vi "save_spectroscopy_hdf.vi"(8 "Spectroscopy cluster in":T1, 11 "file path":path) -> ()   [LabVIEW 2019]
uses:
  <vilib>/UPVI/lvhdf5/file.llb/LVH5F Operation.ctl
  <vilib>/Utility/miscctls.llb/LVRectTypeDef.ctl
  <vilib>/UPVI/lvhdf5/group.llb/H5G_obj_t.ctl
  <vilib>/UPVI/lvhdf5/dataset.llb/LVH5D Operation.ctl
  <vilib>/UPVI/lvhdf5/attribute.llb/LVH5A Operation.ctl
  <vilib>/UPVI/lvhdf5/identifier.llb/Not an HDF5 Refnum Constant.vi
  <vilib>/UPVI/lvhdf5/common.llb/To HDF5 Ref.vi
  global_variables.vi
  <vilib>/UPVI/lvhdf5/attribute.llb/Write Multiple Attributes.vi
  <vilib>/UPVI/lvhdf5/utility.llb/Select HDF5 Dialog.vi
  <vilib>/UPVI/lvhdf5/utility.llb/Select HDF5 Dialog (Object Only).vi
  <vilib>/UPVI/lvhdf5/dataset.llb/Simple H5Dwrite (Variant).vi
  <vilib>/UPVI/lvhdf5/dataset.llb/H5Dclose.vi
  <vilib>/UPVI/lvhdf5/attribute.llb/Simple H5Awrite (Variant).vi
  <vilib>/UPVI/lvhdf5/attribute.llb/LVH5 Write Attributes.xnode
  <vilib>/UPVI/lvhdf5/library.llb/HDF5 Ref.ctl
  <vilib>/UPVI/lvhdf5/dataset.llb/Simple H5Dwrite.xnode
  <vilib>/UPVI/lvhdf5/dataset.llb/Write Dataset with Attributes.xnode
  <vilib>/UPVI/lvhdf5/attribute.llb/Simple H5Awrite.xnode
  <vilib>/Utility/VariantDataType/GetClusterInfo.vi
  <vilib>/Utility/VariantDataType/VariantType.lvlib
  <vilib>/Utility/VariantDataType/GetTypeInfo.vi
  <vilib>/UPVI/lvhdf5/attribute.llb/Cluster to Attribute Array.xnode
  <vilib>/Utility/error.llb/Error Cluster From Error Code.vi
  <vilib>/UPVI/lvhdf5/dataset.llb/OpenCreateReplace Dataset by Element Type.vi
  <vilib>/UPVI/lvhdf5/dataspace.llb/H5Sselect_hyperslab.vi
  <vilib>/UPVI/lvhdf5/dataset.llb/H5Dwrite (Variant).vi
  <vilib>/UPVI/lvhdf5/dataset.llb/H5Dget_space.vi
  <vilib>/UPVI/lvhdf5/attribute.llb/private/LVH5AwriteWDTAttrs.vi
  <vilib>/UPVI/lvhdf5/dataspace.llb/H5Sclose.vi
  <vilib>/UPVI/lvhdf5/utility.llb/Select HDF5 Dialog (File and Object).vi
  <resource>/objmgr/daqmx.rc
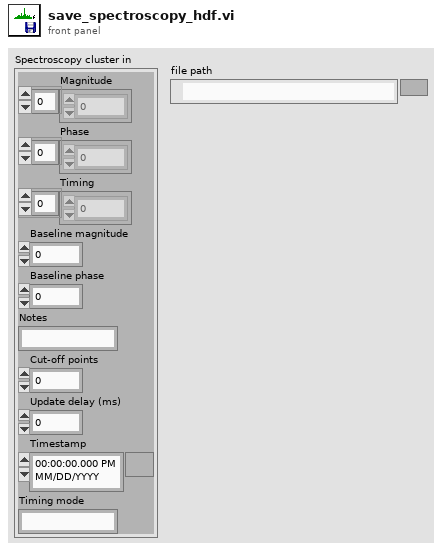
[diagram p1: front panel]
types:
  T1 = cluster{"Magnitude":dbl[], "Phase":dbl[], "Timing":dbl[], "Baseline magnitude":dbl, "Baseline phase":dbl, "Notes":string, "Cut-off points":i32, "Update delay (ms)":dbl, "Timestamp":timestamp, "Timing mode":string}
  T2 = typedef "LVH5F Operation.ctl" = enum16{"open", "open or create", "create or replace", "create or replace (with confirmation)", "create", "open (read only)"}
  T3 = typedef "HDF5 Ref.ctl" = refnum<k1>
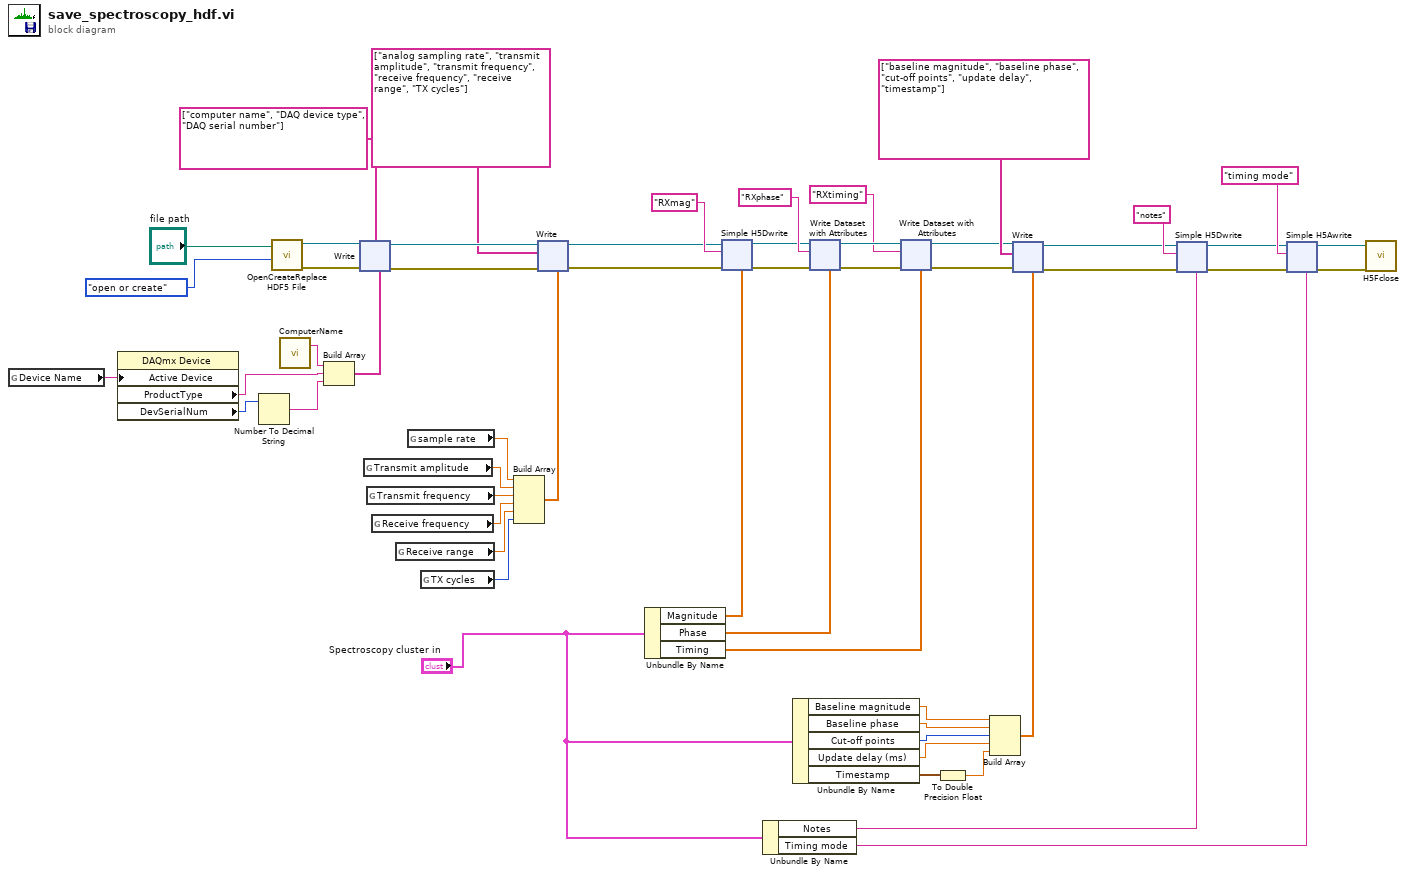
[diagram p0: block diagram]
diagram:
  n1 = global read "global_variables.vi" "Device Name"() -> (w32:tag)
  n2 = property class="DAQmx Device"("Active Device"=w32) -> ("ProductType"=w45:string, "DevSerialNum"=w47:u32)  [unwired: 2 in, 2 out]
  n3 = Number To Decimal String(number=w47) -> (decimal integer string=w46:string)  [unwired: 1 in]
  n4 = call <vilib>:"OpenCreateReplace HDF5 File.vi"("function (open or create)"=LVH5F_Operation."open or create", "path"="file path") -> ("error out"=w30:errorcluster, "HDF5 Ref out"=w31:T3)  [unwired: 6 in]
  n5 = call "ComputerName.vi"() -> ("String/Binary data"=w44:string)  [unwired: 4 in, 1 out]
  n6 = Build Array(w44, w45, w46) -> (w43:string[])
  n7 = xnode "Write"("HDF5 Ref"=w31, "error in (no error)"=w30, "Name(s)"=string[] ["computer name", "DAQ device type", "DAQ serial number"], "Value(s)"=w43) -> ("HDF5 Ref out"=w29:T3, "error out"=w28:errorcluster)  [unwired: 1 in]
  n8 = global read "global_variables.vi" "Transmit amplitude"() -> (w41:dbl)
  n9 = global read "global_variables.vi" "Transmit frequency"() -> (w40:dbl)
  n10 = global read "global_variables.vi" "Receive frequency"() -> (w38:dbl)
  n11 = global read "global_variables.vi" "Receive range"() -> (w37:dbl)
  n12 = global read "global_variables.vi" "sample rate"() -> (w33:dbl)
  n13 = global read "global_variables.vi" "TX cycles"() -> (w36:i32)
  n14 = Build Array(w33, w41, w40, w38, w37, w36) -> (w39:dbl[])
  n15 = xnode "Write"("HDF5 Ref"=w29, "error in (no error)"=w28, "Name(s)"=string[] ["analog sampling rate", "transmit amplitude", "transmit frequency", "receive frequency", "receive range", "TX cycles"], "Value(s)"=w39) -> ("HDF5 Ref out"=w25:T3, "error out"=w26:errorcluster)  [unwired: 1 in]
  n16 = Unbundle By Name("Spectroscopy cluster in") -> ("Magnitude"=w24:dbl[], "Phase"=w23:dbl[], "Timing"=w20:dbl[])
  n17 = xnode "Simple H5Dwrite"("Dataset Path"="RXmag", "error in (no error)"=w26, "HDF5 Path or Ref"=w25, "Data"=w24) -> ("HDF5 Ref out"=w49:T3, "error out"=w50:errorcluster)  [unwired: 4 in, 1 out]
  n18 = Unbundle By Name("Spectroscopy cluster in") -> ("Notes"=w11:string, "Timing mode"=w5:string)
  n19 = Unbundle By Name("Spectroscopy cluster in") -> ("Baseline magnitude"=w16:dbl, "Baseline phase"=w15:dbl, "Cut-off points"=w14:i32, "Update delay (ms)"=w13:dbl, "Timestamp"=w4:timestamp)
  n20 = xnode "Write Dataset with Attributes"("Dataset Path"="RXphase", "error in (no error)"=w50, "HDF5 Path or Ref"=w49, "Data"=w23) -> ("HDF5 Ref out"=w22:T3, "error out"=w21:errorcluster)  [unwired: 4 in, 1 out]
  n21 = xnode "Write Dataset with Attributes"("Dataset Path"="RXtiming", "error in (no error)"=w21, "HDF5 Path or Ref"=w22, "Data"=w20) -> ("HDF5 Ref out"=w18:T3, "error out"=w17:errorcluster)  [unwired: 4 in, 1 out]
  n22 = To Double Precision Float(number=w4) -> (double precision float=w3:dbl)
  n23 = Build Array(w16, w15, w14, w13, w3) -> (w53:dbl[])
  n24 = xnode "Write"("HDF5 Ref"=w18, "error in (no error)"=w17, "Name(s)"=string[] ["baseline magnitude", "baseline phase", "cut-off points", "update delay", "timestamp"], "Value(s)"=w53) -> ("HDF5 Ref out"=w10:T3, "error out"=w9:errorcluster)  [unwired: 1 in]
  n25 = xnode "Simple H5Dwrite"("Dataset Path"="notes", "error in (no error)"=w9, "HDF5 Path or Ref"=w10, "Data"=w11) -> ("HDF5 Ref out"=w7:T3, "error out"=w6:errorcluster)  [unwired: 4 in, 1 out]
  n26 = xnode "Simple H5Awrite"("HDF5 Ref"=w7, "Name"="timing mode", "error in (no error)"=w6, "Value"=w5) -> ("HDF5 Ref out"=w2:T3, "error out"=w1:errorcluster)  [unwired: 1 in]
  n27 = call <vilib>:"H5Fclose.vi"("error in (no error)"=w1, "HDF5 Ref"=w2) -> ()  [unwired: 7 in, 1 out]
